vi "Lockin check on.vi"(11 "VISA resource name":refnum<visa-resource-name>="GPIB0::9::INSTR") -> (2 "ready?":bool, 3 "VISA resource name out":refnum<visa-resource-name>)   [LabVIEW 2009, in "Lockin.lvclass"]
doc: "Checks to see if the SR830 lock-in amplifier is available or not by requesting its device ID string."
uses:
  Lockin.lvclass
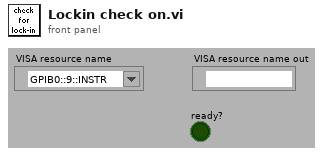
[diagram p1: front panel]
types:
  T1 = typedef "Semaphore RefNum" = refnum<k1>
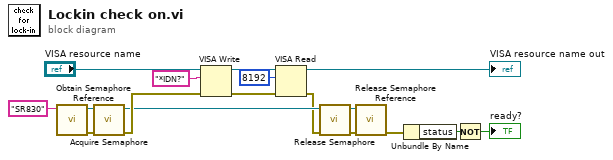
[diagram p0: block diagram]
diagram:
  n1 = call <vilib>:"Obtain Semaphore Reference.vi"("name (unnamed)"="SR830") -> ("error out"=w10:errorcluster, "semaphore"=w9:T1)  [unwired: 2 in, 3 out]
  n2 = call <vilib>:"Acquire Semaphore.vi"("error in (no error)"=w10, "semaphore"=w9) -> ("error out"=w8:errorcluster, "semaphore out"=w5:T1)  [unwired: 1 in, 3 out]
  n3 = VISA Write(VISA resource name="VISA resource name", write buffer="*IDN?" ("data"), error in (no error)=w8) -> (VISA resource name out=w12:refnum<visa-resource-name>, error out=w11:errorcluster)  [unwired: 1 out]
  n4 = VISA Read(VISA resource name=w12, byte count=8192, error in (no error)=w11) -> (VISA resource name out=→"VISA resource name out":refnum<visa-resource-name>, error out=w4:errorcluster)  [unwired: 2 out]
  n5 = call <vilib>:"Release Semaphore.vi"("error in (no error)"=w4, "semaphore"=w5) -> ("error out"=w7:errorcluster, "semaphore out"=w6:T1)  [unwired: 4 out]
  n6 = call <vilib>:"Release Semaphore Reference.vi"("error in (no error)"=w7, "semaphore"=w6) -> ("error out"=w3:errorcluster)  [unwired: 9 out]
  n7 = Unbundle By Name(w3) -> ("status"=w17:bool)
  n8 = Not(x=w17) -> (.not. x?=→"ready?":bool)
